vi "ingest.avro_stream_new_dataset.vi"(8 "error in":errorcluster, 11 "DatasetCreateStaging in":refnum<class "DatasetCreateStaging.lvclass">) -> (0 "error out":errorcluster, 3 "DatasetCreateStaging out":refnum<class "DatasetCreateStaging.lvclass">)   [LabVIEW 2020, in "DatasetCreateStaging.lvclass"]
doc: "Ingests a Nominal Avro-stream file into a newly created dataset."
uses:
  DatasetCreateStaging.lvclass
  DatasetCreateStaging.lvclass/DatasetCreateStaging.ctl
  client.lvlib
panel:
  out "out_job out":i32
  in  "file_path":string
  in  "dataset_create":i32
  in  "out_job":i32
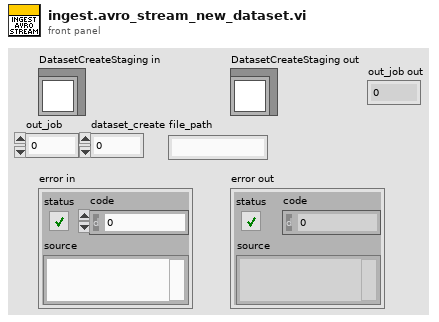
[diagram p1: front panel]
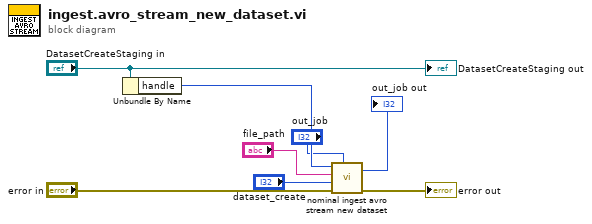
[diagram p0: block diagram]
diagram:
  n1 = Unbundle By Name("DatasetCreateStaging in") -> ("handle"=w6:i32)
  n2 = call "nominal ingest avro stream new dataset.vi"("out_job"="out_job", "error in (no error)"="error in", "dataset_create"="dataset_create", "file_path"="file_path", "client"=w6) -> ("error out"=→"error out":errorcluster, "out_job out"=→"out_job out":i32)  [unwired: 4 in, 1 out]
  "DatasetCreateStaging out" <- "DatasetCreateStaging in"
